vi "Create Shared Variable.vi"(8 "error in (no error)":errorcluster, 9 "data type":T1(ring)=enum."double", 10 "shared variable name":string="my_number", 11 "process name out":string="sv_alarm_example") -> (0 "error out":errorcluster, 3 "shared variable":refnum<k21>="\\\\.\\sv_alarm_example\\my_number")   [LabVIEW 2018, in "Dynamic Shared Variables.lvlib"]
doc: "Creates an IO Shared Variable"
uses:
  Dynamic Shared Variables.lvlib
  <vilib>/lvdsc/NI_DSC.lvlib
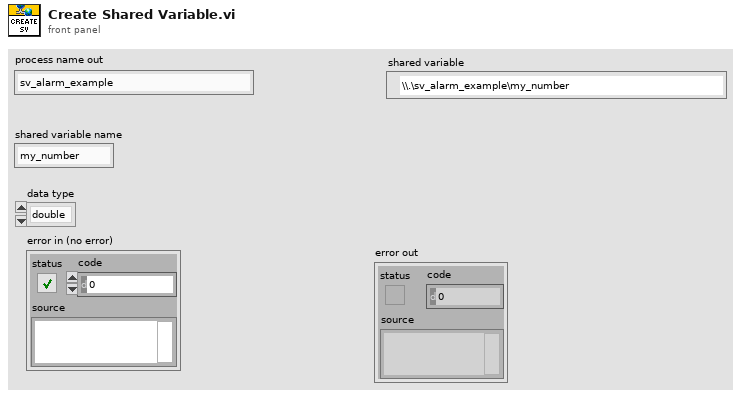
[diagram p1: front panel]
types:
  T1 = enum32{"u32BitField", "bool", "double", "string", "int8", "uint8", "int16", "uint16", "int32", "uint32", "int64", "uint64", "single", "double waveform", "int16 waveform", "array of boolean", "array of int8", "array of uint8", "array of int16", "array of uint16", "array of int32", "array of uint32", "array of int64", "array of uint64", "array of single", "array of double", "array of double waveform", "array of int16 waveform", "array of string", "variant", "timestamp", "fixed point", "custom"}
  T2 = cluster{"use binding? (F)":bool, "URL":string, "access type":enum32{"Read only", "Write only", "Read/write"}, "buffer size":u32, "use buffering? (F)":bool, "single writer? (F)":bool}
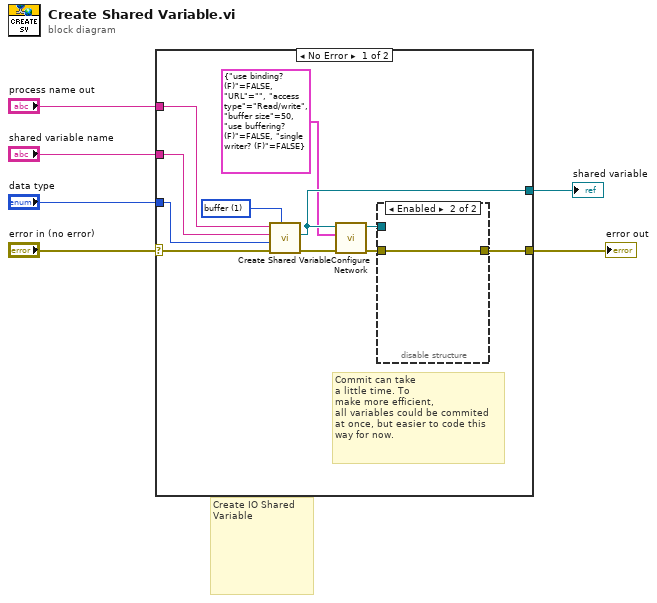
[diagram p0: block diagram]
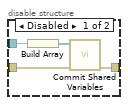
[diagram p2: hidden frame]
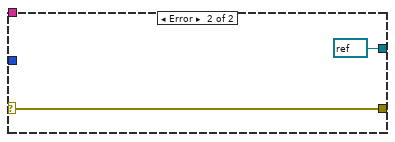
[diagram p3: hidden frame]
diagram:
  # "Create IO Shared Variable"
  n1 = case shown="No Error" "error in (no error)" {
    selector: "error in (no error)" -> [w10 w24]
    tunnel: "shared variable name" -> [w16 _]
    tunnel: "data type" -> [w15 _]
    tunnel: [w14 refnum<k21> refnum ("shared variable")] -> w4
    tunnel: "process name out" -> [w11 _]
    tunnel: [w8 w24] -> w2
    frame No Error {
      w17 = u16 1 items=["commit", "buffer"] ("set mode")
      # "Commit can take\na little time. To\nmake more efficient,\nall variables could be commited\nat once, but easier to code this\nway for now."
      n2 = call <vilib>:"Create Shared Variable.vi"("set mode"=w17, "error in (no error)"=w10, "data type"=w15, "shared variable name"=w16, "process name"=w11) -> ("error out"=w13:errorcluster, "shared variable"=w14:refnum<k21>)  [unwired: 4 in, 1 out]
      n3 = call <vilib>:"Configure Network.vi"("error in (no error)"=w13, "network settings"=T2 {"use binding? (F)"=FALSE, "URL"="", "access type"=enum."Read/write", "buffer size"=50, "use buffering? (F)"=FALSE, "single writer? (F)"=FALSE}, "variable reference in"=w14) -> ("error out"=w9:errorcluster, "variable reference out"=w7:refnum<k21>)  [unwired: 7 in]
      n4 = disable-structure shown="Enabled" {
        disable-tunnel: w9 -> [w20 w22]
        disable-tunnel: [w19 w22] -> w8
        disable-tunnel: w7 -> [w18 _]
        frame Disabled {
          n5 = Build Array(w18) -> (w21:refnum<k21>[])
          n6 = call <vilib>:"Commit Shared Variables.vi"("error in (no error)"=w20, "shared variables"=w21) -> ("error out"=w19:errorcluster)  [unwired: 8 in, 1 out]
        }
        frame Enabled {
        }
      }
    }
    frame Error {
    }
  }
  "error out" <- w2
  "shared variable" <- w4
